vi "ZMQ Sine Wave Client for PI.vi"() -> ()   [LabVIEW 2014]
uses:
  <vilib>/addons/zeromq/socket_type.ctl
  <vilib>/addons/zeromq/zmq_context.lvclass
  <vilib>/addons/zeromq/zmq_socket.lvclass
  <vilib>/addons/zeromq/zeromq.lvlib
panel:
  out "LVled":bool
  out "z":dbl
  out "y":dbl
  out "Angle":i32
  in  "LVbtn":bool
  out "Waveform Chart":T1(graph)={"[0]"=1.251, "[1]"=1.095, "[2]"=0.0, "[3]"=0.0, "[4]"=0.0, "[5]"=0.0, "[6]"=0.0, "[7]"=0.0, "[8]"=0.0}
  out "data":string="Hello !!!"
  out "error out":errorcluster
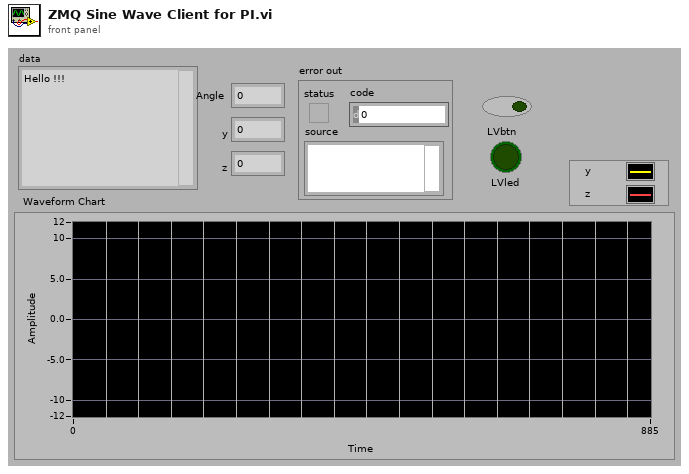
[diagram p1: front panel]
types:
  T1 = cluster{"[0]":dbl, "[1]":dbl, "[2]":dbl, "[3]":dbl, "[4]":dbl, "[5]":dbl, "[6]":dbl, "[7]":dbl, "[8]":dbl}
  T2 = cluster{"[0]":dbl, "[1]":dbl, "[2]":dbl, "[3]":dbl, "[4]":dbl, "[5]":dbl, "[6]":dbl, "[7]":dbl, "[8]":dbl}[]
  T3 = typedef "zeromq.lvlib/socket_type.ctl" = enum8{"ZMQ_PAIR", "ZMQ_PUB", "ZMQ_SUB", "ZMQ_REQ", "ZMQ_REP", "ZMQ_DEALER", "ZMQ_ROUTER", "ZMQ_PULL", "ZMQ_PUSH", "ZMQ_XPUB", "ZMQ_XSUB"}
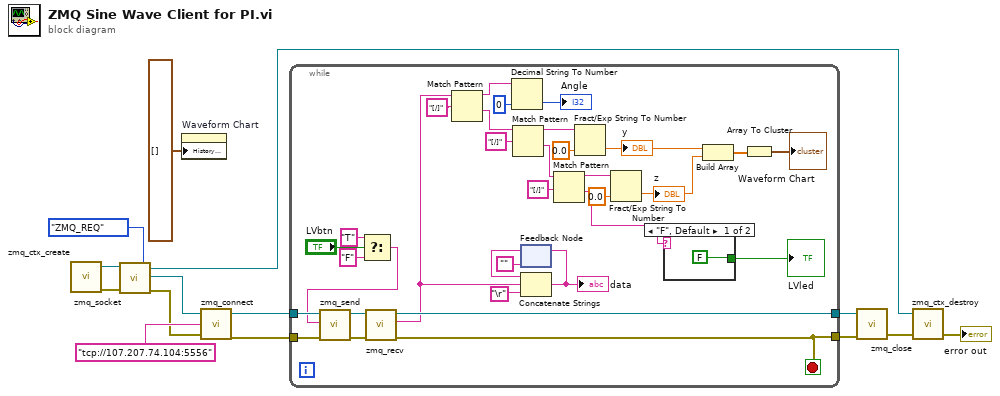
[diagram p0: block diagram]
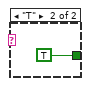
[diagram p2: hidden frame]
diagram:
  n1 = call <vilib>:"zmq_ctx_create.vi"() -> ("error out"=w13:errorcluster, "context out"=w14:refnum<class "zmq_context.lvclass">)  [unwired: 4 in]
  n2 = call <vilib>:"zmq_socket.vi"("error in"=w13, "socket type"=socket_type."ZMQ_REQ", "context in"=w14) -> ("error out"=w9:errorcluster, "socket out"=w11:refnum<class "zmq_socket.lvclass">, "context out"=w6:refnum<class "zmq_context.lvclass">)  [unwired: 2 in]
  n3 = property on="Waveform Chart" class="WFChart (strict)"("History Data"=T2 []) -> ()  [unwired: 2 in, 2 out]
  n4 = call <vilib>:"zmq_connect.vi"("error in"=w9, "endpoint"="tcp://107.207.74.104:5556" ("TCP address"), "socket in"=w11) -> ("error out"=w3:errorcluster, "socket out"=w4:refnum<class "zmq_socket.lvclass">)  [unwired: 1 in]
  n5 = while {
    tunnel: w3 -> [w46]
    tunnel: [w43] -> w8
    tunnel: w4 -> [w47]
    tunnel: [w42] -> w2
    stop <- w43 stop-if-true
    n6 = Select(t="T", s="LVbtn", f="F") -> (s? t:f=w38:string)
    n7 = call <vilib>:"zmq_send.vi"("error in"=w46, "data"=w38, "socket in"=w47) -> ("error out"=w44:errorcluster, "socket out"=w45:refnum<class "zmq_socket.lvclass">)  [unwired: 4 in]
    n8 = call <vilib>:"zmq_recv.vi"("error in"=w44, "socket in"=w45) -> ("error out"=w43:errorcluster, "data"=w22:string, "socket out"=w42:refnum<class "zmq_socket.lvclass">)  [unwired: 3 in, 2 out]
    n9 = Match Pattern(string=w22, regular expression="[/]") -> (before substring=w36:string, after substring=w32:string)  [unwired: 1 in, 2 out]
    n10 = Decimal String To Number(string=w36, default (0L)=0 ("default (0 I32)")) -> (number=→"Angle":i32)  [unwired: 1 in, 1 out]
    n11 = Match Pattern(string=w32, regular expression="[/]") -> (before substring=w31:string, after substring=w28:string)  [unwired: 1 in, 2 out]
    n12 = feedback #1("") -> (w25:string)
    n13 = Concatenate Strings(w25, w22, "\r") -> (w23:string)
    "data" <- w23
    n14 = feedback-in #1(w23) -> ()
    n15 = Match Pattern(string=w28, regular expression="[/]") -> (before substring=w30:string, after substring=w15:string)  [unwired: 1 in, 2 out]
    n16 = Fract/Exp String To Number(string=w31, default (0 dbl)=0.0 ("default (0 I32)")) -> (number=w20:dbl)  [unwired: 2 in, 1 out]
    "y" <- w20
    n17 = Fract/Exp String To Number(string=w30, default (0 dbl)=0.0 ("default (0 I32)")) -> (number=w19:dbl)  [unwired: 2 in, 1 out]
    "z" <- w19
    n18 = case shown="\"F\", Default" w15 {
      tunnel: [FALSE TRUE] -> w16
      frame "F", Default {
      }
      frame "T" {
      }
    }
    "LVled" <- w16
    n19 = Build Array(w20, w19) -> (w18:dbl[])
    n20 = Array To Cluster(array=w18) -> (cluster=→"Waveform Chart":T1)
  }
  n21 = call <vilib>:"zmq_close.vi"("error in"=w8, "socket"=w2) -> ("error out"=w7:errorcluster)  [unwired: 3 in]
  n22 = call <vilib>:"zmq_ctx_destroy.vi"("error in"=w7, "context in"=w6) -> ("error out"=→"error out":errorcluster)  [unwired: 3 in]
